vi "Write Channels to scan.vi"(8 "error in (no error)":errorcluster, 9 "Seconds between samples":dbl=1.0 format="%_4f", 10 "Channels to scan (empty - don't use scanner option)":i32[](array[numeric]), 11 "Instrument with scanner.lvclass in":refnum<class "Instrument with scanner.lvclass">) -> (0 "error out":errorcluster, 3 "Instrument with scanner.lvclass out":refnum<class "Instrument with scanner.lvclass">)   [LabVIEW 2015, in "Instrument with scanner.lvclass"]
uses:
  Instrument with scanner.lvclass
  Instrument with scanner.lvclass/Instrument with scanner.ctl
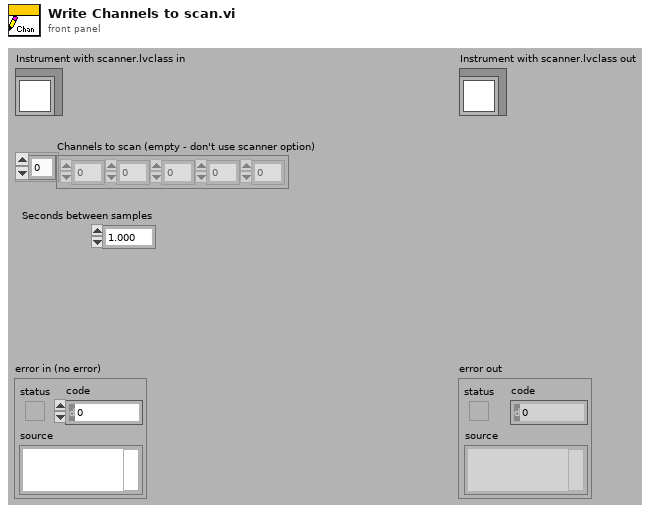
[diagram p1: front panel]
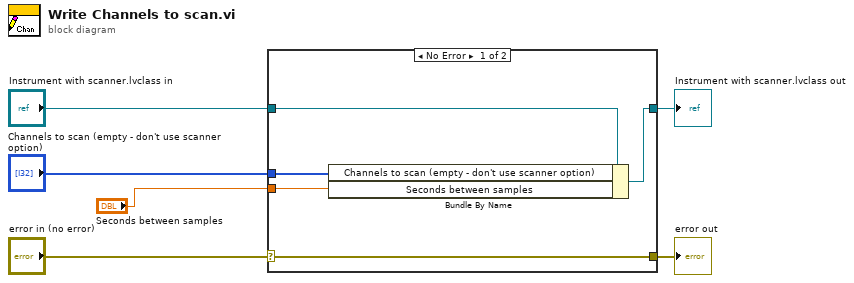
[diagram p0: block diagram]
diagram:
  n1 = case shown="No Error" "error in (no error)" {
    selector: "error in (no error)" -> [w11 w12]
    tunnel: [w11 w12] -> w5
    tunnel: [w9 w13] -> w3
    tunnel: "Instrument with scanner.lvclass in" -> [w10 w13]
    tunnel: "Channels to scan (empty - don't use scanner option)" -> [w8 _]
    tunnel: "Seconds between samples" -> [w7 _]
    frame No Error {
      n2 = Bundle By Name(cluster=w10, "Channels to scan (empty - don't use scanner option)"=w8, "Seconds between samples"=w7) -> (w9:refnum<class "Instrument with scanner.lvclass">)
    }
    frame Error {
    }
  }
  "error out" <- w5
  "Instrument with scanner.lvclass out" <- w3
